vi "纳清_手动清洗.vi"(7 "探头":T1(ring), 8 "error in (no error)":errorcluster caption="错误输入（无错误）") -> (0 "error out":errorcluster caption="错误输出")   [LabVIEW 2016, in "斯坦道多参数.lvlib"]
uses:
  <vilib>/Plasmionique/MB Master/MB_Master/MB_Master.lvclass
  <vilib>/Plasmionique/MB Master/MB Master.lvlib
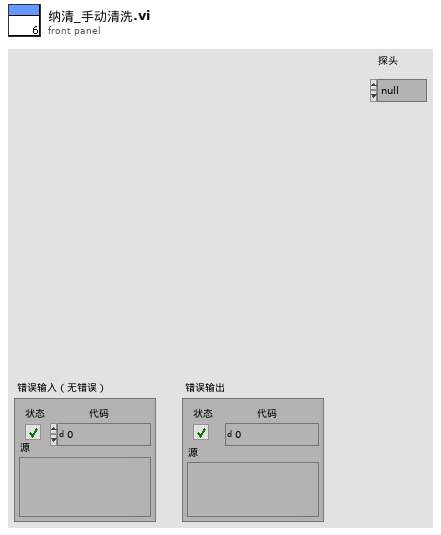
[diagram p1: front panel]
types:
  T1 = enum16{"null", "pH", "DO", "浊度", "电导率", "叶绿素a", "藻密度"}
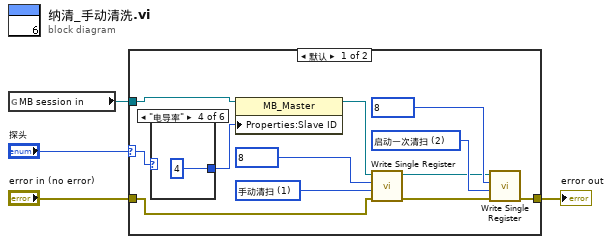
[diagram p0: block diagram]
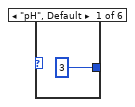
[diagram p2: hidden frame]
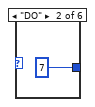
[diagram p3: hidden frame]
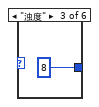
[diagram p4: hidden frame]
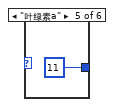
[diagram p5: hidden frame]
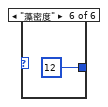
[diagram p6: hidden frame]
diagram:
  n1 = global read "多参数全局变量.vi" "MB session in"() -> (w1:refnum<class "MB_Master.lvclass">)
  n2 = case shown="默认" "探头" {
    selector: "探头" -> [w12 _]
    tunnel: "error in (no error)" -> [w10 w23]
    tunnel: [w16 w23] -> w3
    tunnel: w1 -> [w15 _]
    frame Default {
      w5 = u16 1 items=["自动清扫", "手动清扫", "启动一次清扫"] ("清扫模式")
      w11 = u16 2 items=["自动清扫", "手动清扫", "启动一次清扫"] ("清扫模式")
      n3 = case shown="\"电导率\"" w12 {
        tunnel: [3 7 8 4 11 12] -> w14
        frame "pH", Default {
        }
        frame "DO" {
        }
        frame "浊度" {
        }
        frame "电导率" {
        }
        frame "叶绿素a" {
        }
        frame "藻密度" {
        }
      }
      n4 = property class="MB_Master"(reference=w15, "Properties:Slave ID"=w14) -> (reference out=w8:refnum<class "MB_Master.lvclass">)  [unwired: 1 in, 1 out]
      n5 = call <vilib>:"Write Single Register.vi"("error in (no error)"=w10, "value"=w5, "address"=u16 8 ("starting address"), "MB session in"=w8) -> ("error out"=w9:errorcluster, "MB session out"=w7:refnum<class "MB_Master.lvclass">)  [unwired: 6 in]
      n6 = call <vilib>:"Write Single Register.vi"("error in (no error)"=w9, "value"=w11, "address"=u16 8 ("starting address"), "MB session in"=w7) -> ("error out"=w16:errorcluster)  [unwired: 6 in, 1 out]
    }
    frame "null" {
    }
  }
  "error out" <- w3
